vi "Impulse Pattern.vi"(2 "delay":i32, 3 "amplitude":dbl=1.0 format="%0.2f", 4 "samples":i32=128) -> (0 "error":i32, 1 "Impulse Pattern":dbl[](array[numeric]))   [LabVIEW 2017, in "NI_AALBase.lvlib"]
doc: "Generates an array containing an impulse pattern."
uses:
  NI_AALBase.lvlib
  lvanlys.dll
panel:
  # "Impulse Pattern"
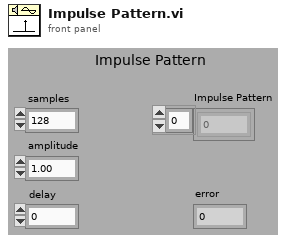
[diagram p1: front panel]
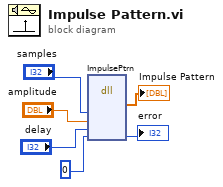
[diagram p0: block diagram]
diagram:
  n1 = dll-call lib="C:/Program Files/National Instruments/LabVIEW 2017/resource/lvanlys.*" fn="ImpulsePtrn"("samples"="samples", "amplitude"="amplitude", "delay"="delay", 0) -> ("Impulse Pattern"=→"Impulse Pattern":dbl[], →"error":i32)  [unwired: 8 in, 2 out]
